vi "Manage Sound Eff Events.vi"(7 "event":enum16{"Play", "Stop"}(ring), 8 "error in (no error)":errorcluster, 9 "path":path, 10 "Sound Effect Off":T1, 11 "Sounds In":cluster{"Sound Effect":T1, "Task ID":T2}[](array[cluster]) {"Task ID" format="%.0x"}) -> (0 "error out":errorcluster, 3 "Sounds out":cluster{"Sound Effect":T1, "Task ID":T2}[](array[cluster]) {"Task ID" format="%.0x"})   [LabVIEW 2021, in "Application.lvclass"]
uses:
  Application.lvclass
  Sound Effects.ctl
  <vilib>/sound2/lvsound2.llb/Sound Output Task ID.ctl
  <vilib>/sound2/lvsound2.llb/Sound Output Set Volume (Single).vi
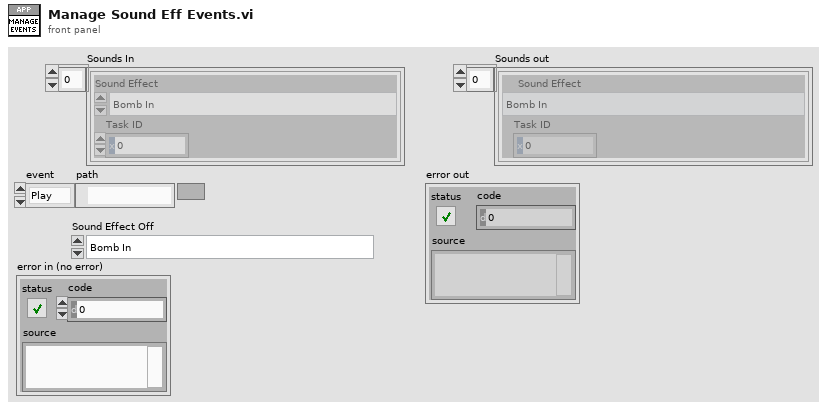
[diagram p1: front panel]
types:
  T1 = typedef "Application.lvclass/Sound Effects.ctl" = enum16{"Bomb In", "Bomb Out", "Bomb Touched", "Game Over", "Victory", "Eat", "10 Fruits", "Eat2", "Eat3", "Eat4", "MaxShield", "Shield", "10p", "Grape In", "Grape Out", "20p", "30p", "40p", "50p", "60p", "70p", "80p", "90p", "100p", "All shields cracked", "Mouse In", "Mouse Out", "Mouse Eaten", "Grape Eaten", "States Recover", "Broken Shield", "Bonus", "Happy Time", "explode", "Game over musica", "Back Music", "Shield Catch", "Evil lough", "Cricket In", "Cricket eaten", "Lets Go", "Jump1", "Jump2", "Jump3", "Unstoppable", "Troll Music", "winner"}
  T2 = typedef "Sound Output Task ID.ctl" = u32
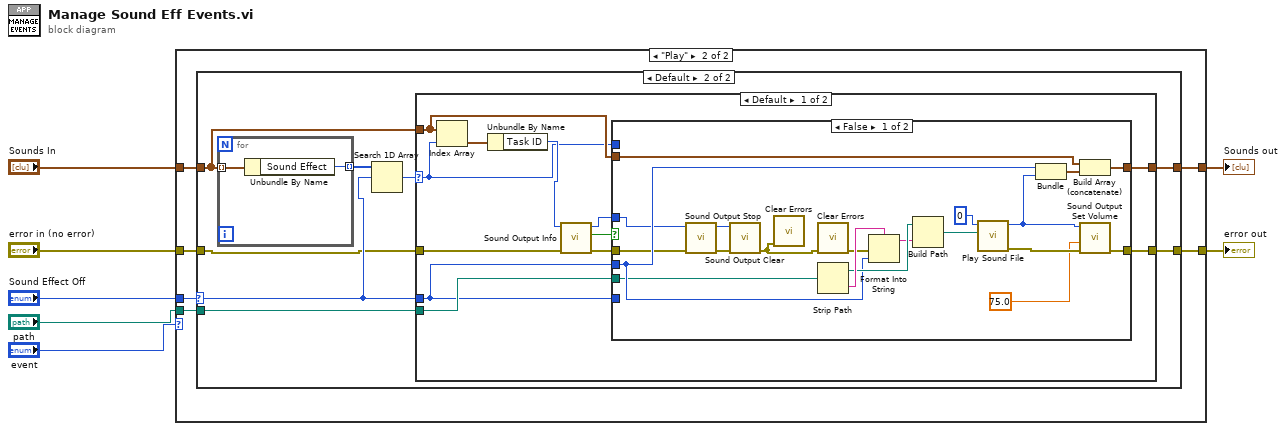
[diagram p0: block diagram]
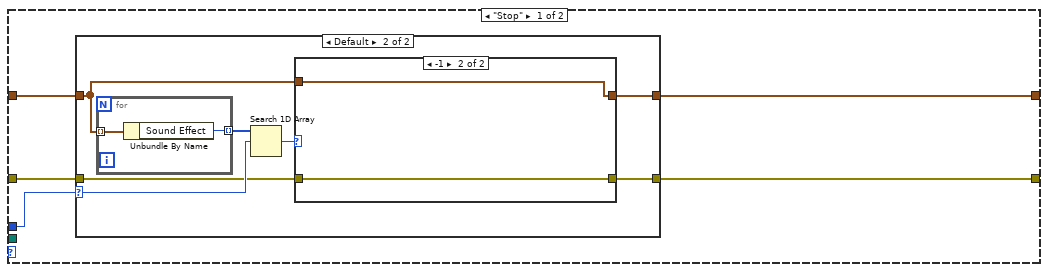
[diagram p2: hidden frame]
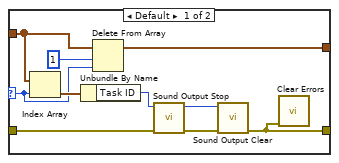
[diagram p4: hidden frame]
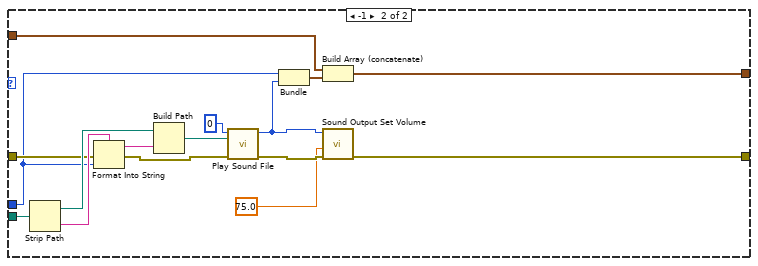
[diagram p7: hidden frame]
diagram:
  n1 = case shown="\"Play\"" "event" {
    tunnel: [w12 w41] -> w7
    tunnel: "Sounds In" -> [w11 w40]
    tunnel: "Sound Effect Off" -> [w10 w39]
    tunnel: "path" -> [_ w38]
    tunnel: [w8 w37] -> w1
    tunnel: "error in (no error)" -> [w9 w36]
    frame "Stop" {
      n2 = case shown="Default" w10 {
        selector: w10 -> [_ w21]
        tunnel: w11 -> [w14 w18]
        tunnel: [w14 w17] -> w12
        tunnel: w9 -> [w13 w16]
        tunnel: [w13 w15] -> w8
        frame "Back Music" {
        }
        frame Default {
          n3 = for {
            tunnel: w18 -> [w35] mode=indexing
            tunnel: [w34] -> w20 mode=indexing
            n4 = Unbundle By Name(w35) -> ("Sound Effect"=w34:T1)
          }
          n5 = Search 1D Array(1D array=w20, element=w21) -> (index of element=w19:i32)  [unwired: 1 in]
          n6 = case shown="-1" w19 {
            selector: w19 -> [w25 _]
            tunnel: w18 -> [w27 w33]
            tunnel: [w24 w33] -> w17
            tunnel: w16 -> [w23 w32]
            tunnel: [w22 w32] -> w15
            frame Default {
              n7 = Index Array(array=w27, index=w25) -> (element=w31:cluster{"Sound Effect":T1, "Task ID":T2})
              n8 = Unbundle By Name(w31) -> ("Task ID"=w30:T2)
              n9 = Delete From Array(array=w27, length=1, index=w25) -> (array with subset deleted=w24:cluster{"Sound Effect":T1, "Task ID":T2}[])  [unwired: 1 out]
              n10 = call <vilib>:"Sound Output Stop.vi"("error in (no error)"=w23, "task ID"=w30) -> ("error out"=w28:errorcluster, "task ID out"=w29:T2)  [unwired: 8 in]
              n11 = call <vilib>:"Sound Output Clear.vi"("error in (no error)"=w28, "task ID"=w29) -> ("error out"=w22:errorcluster)  [unwired: 9 in]
              n12 = call <vilib>:"Clear Errors.vi"("error in (no error)"=w22) -> ()  [unwired: 5 in, 2 out]
            }
            frame -1 {
            }
          }
        }
      }
    }
    frame "Play" {
      n13 = case shown="Default" w39 {
        selector: w39 -> [_ w47]
        tunnel: w40 -> [w43 w49]
        tunnel: [w43 w48] -> w41
        tunnel: w38 -> [_ w46]
        tunnel: [w42 w45] -> w37
        tunnel: w36 -> [w42 w44]
        frame "Back Music" {
        }
        frame Default {
          n14 = for {
            tunnel: w49 -> [w103] mode=indexing
            tunnel: [w102] -> w51 mode=indexing
            n15 = Unbundle By Name(w103) -> ("Sound Effect"=w102:T1)
          }
          n16 = Search 1D Array(1D array=w51, element=w47) -> (index of element=w50:i32)  [unwired: 1 in]
          n17 = case shown="Default" w50 {
            selector: w50 -> [w58 _]
            tunnel: w49 -> [w60 w92]
            tunnel: [w59 w91] -> w48
            tunnel: w47 -> [w52 w86]
            tunnel: w46 -> [w55 w90]
            tunnel: [w54 w89] -> w45
            tunnel: w44 -> [w53 w88]
            frame Default {
              n18 = Index Array(array=w60, index=w58) -> (element=w63:cluster{"Sound Effect":T1, "Task ID":T2})
              n19 = Unbundle By Name(w63) -> ("Task ID"=w62:T2)
              n20 = call <vilib>:"Sound Output Info.vi"("error in (no error)"=w53, "task ID"=w62) -> ("error out"=w56:errorcluster, "is playing?"=w61:bool, "task ID out"=w57:T2)  [unwired: 6 in, 1 out]
              n21 = case shown="False" w61 {
                tunnel: w60 -> [w76 w85]
                tunnel: [w75 w85] -> w59
                tunnel: w58 -> [_ _]
                tunnel: w57 -> [w69 _]
                tunnel: w56 -> [w68 w84]
                tunnel: w52 -> [w73 _]
                tunnel: w55 -> [w72 _]
                tunnel: [w66 w84] -> w54
                tunnel: w52 -> [_ _]
                frame False {
                  n22 = call <vilib>:"Sound Output Stop.vi"("error in (no error)"=w68, "task ID"=w69) -> ("error out"=w70:errorcluster, "task ID out"=w71:T2)  [unwired: 8 in]
                  n23 = call <vilib>:"Sound Output Clear.vi"("error in (no error)"=w70, "task ID"=w71) -> ("error out"=w67:errorcluster)  [unwired: 9 in]
                  n24 = call <vilib>:"Clear Errors.vi"("error in (no error)"=w67) -> ()  [unwired: 5 in, 2 out]
                  n25 = call <vilib>:"Clear Errors.vi"("error in (no error)"=w67) -> ("error out"=w65:errorcluster)  [unwired: 5 in, 1 out]
                  n26 = Strip Path(path=w72) -> (stripped path=w80:path, name=w81:string)
                  n27 = Format Into String(format string=w81, error in=w65, w73) -> (resulting string=w79:string)  [unwired: 1 in, 1 out]
                  n28 = Build Path(base path=w80, name or relative path=w79) -> (appended path=w78:path)
                  n29 = call <vilib>:"Play Sound File.vi"("path"=w78, "device ID"=u32 0) -> ("error out"=w82:errorcluster, "task ID"=w77:T2)  [unwired: 8 in]
                  n30 = Bundle("Sound Effect Off"=w73, "task ID"=w77) -> (w74:cluster{"Sound Effect Off":T1, "task ID":T2})  [unwired: 1 in]
                  n31 = Build Array (concatenate)(w76, w74) -> (w75:cluster{"Sound Effect Off":T1, "task ID":T2}[])
                  n32 = call-poly <vilib>:"Sound Output Set Volume.vi"("error in (no error)"=w82, "volume"=75.0, "task ID"=w77) -> ("error out"=w66:errorcluster)  [unwired: 7 in, 1 out]
                }
                frame True {
                }
              }
            }
            frame -1 {
              n33 = Strip Path(path=w90) -> (stripped path=w97:path, name=w98:string)
              n34 = Format Into String(format string=w98, error in=w88, w86) -> (resulting string=w96:string, error out=w87:errorcluster)  [unwired: 1 in]
              n35 = Build Path(base path=w97, name or relative path=w96) -> (appended path=w95:path)
              n36 = call <vilib>:"Play Sound File.vi"("error in (no error)"=w87, "path"=w95, "device ID"=u32 0) -> ("error out"=w100:errorcluster, "task ID"=w94:T2)  [unwired: 7 in]
              n37 = Bundle("Sound Effect Off"=w86, "task ID"=w94) -> (w93:cluster{"Sound Effect Off":T1, "task ID":T2})  [unwired: 1 in]
              n38 = Build Array (concatenate)(w92, w93) -> (w91:cluster{"Sound Effect Off":T1, "task ID":T2}[])
              n39 = call-poly <vilib>:"Sound Output Set Volume.vi"("error in (no error)"=w100, "volume"=75.0, "task ID"=w94) -> ("error out"=w89:errorcluster)  [unwired: 7 in, 1 out]
            }
          }
        }
      }
    }
  }
  "Sounds out" <- w7
  "error out" <- w1
